vi "Perform Step.vi"(8 "error in (no error)":errorcluster, 11 "Disabled Assertion in":refnum<class "Disabled Assertion.lvclass">) -> (0 "error out":errorcluster, 2 "Result":T1, 3 "Disabled Assertion out":refnum<class "Disabled Assertion.lvclass">)   [LabVIEW 2020, in "MacroAssert.lvlib" / "Disabled Assertion.lvclass"]
uses:
  Disabled Assertion.lvclass
  Disabled Assertion.lvclass/Disabled Assertion.ctl
  MacroAssert.lvlib
  CTLs/Report Data.ctl
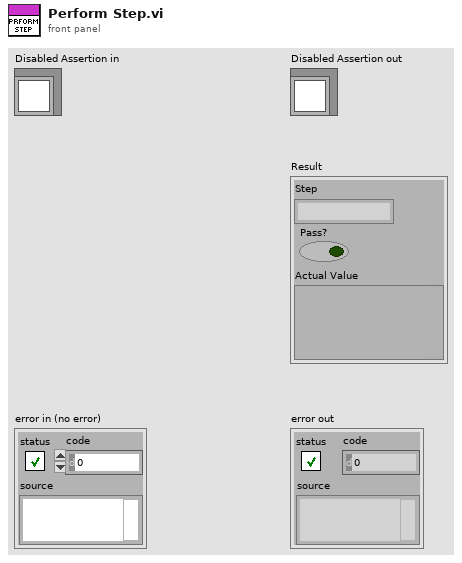
[diagram p1: front panel]
types:
  T1 = typedef "MacroAssert.lvlib/Report Data.ctl" = cluster{"Step":string, "Pass?":bool, "Actual Value":variant}
  T2 = enum8{"Enabled", "Disabled", "Disabled and Grayed Out"}
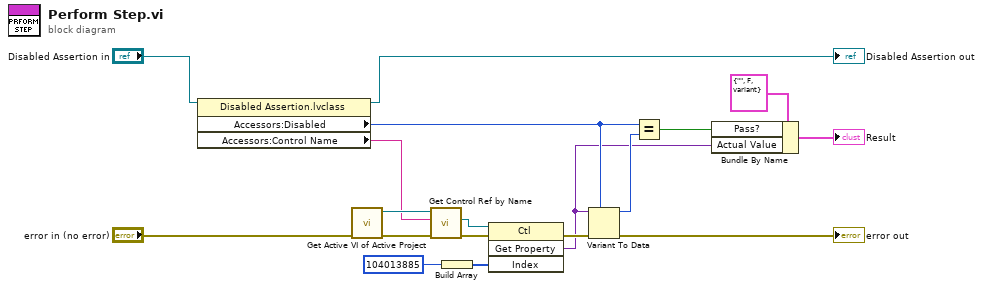
[diagram p0: block diagram]
diagram:
  n1 = property class="Disabled Assertion.lvclass"(reference="Disabled Assertion in") -> (reference out=→"Disabled Assertion out":refnum<class "Disabled Assertion.lvclass">, "Accessors:Disabled"=w5:T2, "Accessors:Control Name"=w6:string)  [unwired: 1 in, 1 out]
  n2 = call "Get Active VI of Active Project.vi"("error in (no error)"="error in (no error)") -> ("error out"=w18:errorcluster, "Active VI Ref"=w17:refnum<vi>)  [unwired: 9 in]
  n3 = call "Get Control Ref by Name.vi"("error in (no error)"=w18, "Name"=w6, "VI Ref"=w17) -> ("error out"=w13:errorcluster, "Ctl Ref"=w9:refnum<vi>)  [unwired: 6 in, 1 out]
  n4 = Build Array(104013885) -> (w11:i32[])
  n5 = invoke class="Ctl" method="Get Property"(reference=w9, error in=w13, "Index"=w11) -> (error out=w14:errorcluster, "GetProperty"=w2:variant)  [unwired: 1 in, 2 out]
  n6 = Variant To Data(error in=w14, type=w5, Variant=w2) -> (data=w10:T2, error out=→"error out":errorcluster)
  n7 = Equal?(x=w5, y=w10) -> (x = y?=w3:bool)
  n8 = Bundle By Name(cluster=T1 {"Step"="", "Pass?"=FALSE, "Actual Value"=variant} ("Report Data"), "Pass?"=w3, "Actual Value"=w2) -> (→"Result":T1)
